vi "SaveParameters.vi"(9 "JSON_Text":string, 11 "ShiftConfigPath":path) -> ()   [LabVIEW 2017]
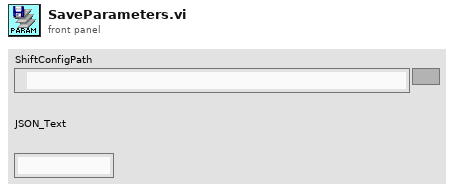
[diagram p1: front panel]
types:
  T1 = enum16{"open", "replace", "create", "open or create", "replace or create", "replace or create with confirmation"}
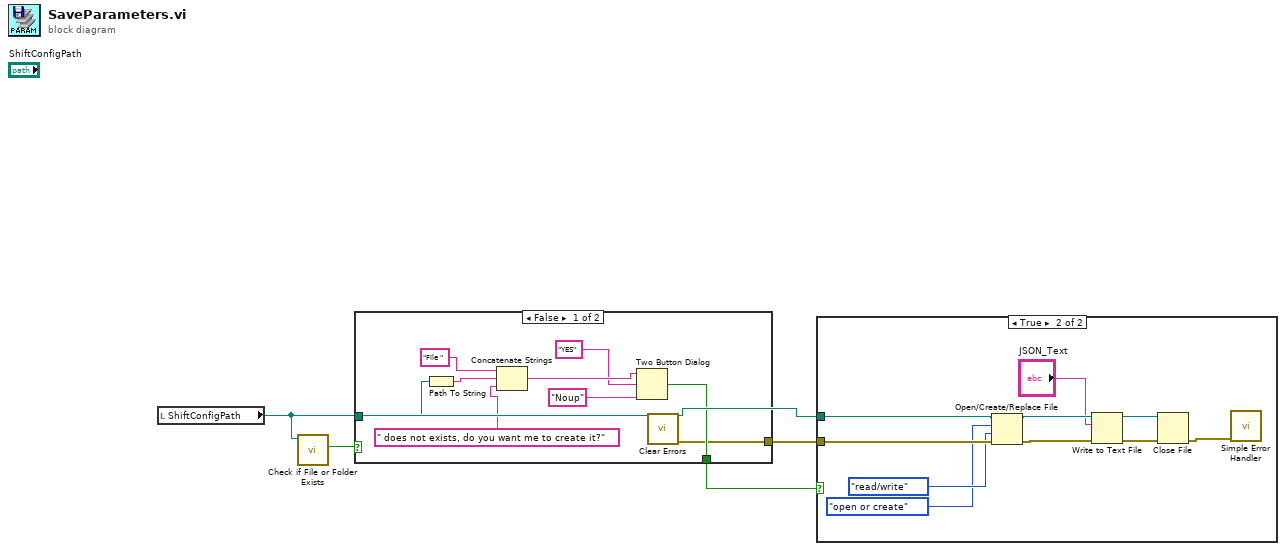
[diagram p0: block diagram]
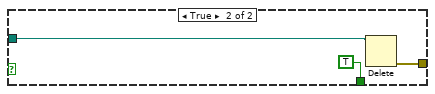
[diagram p3: hidden frame]
diagram:
  n1 = local read "ShiftConfigPath"() -> (w3:path)
  n2 = call <vilib>:"Check if File or Folder Exists.vi"("path"=w3) -> ("file or folder exists?"=w2:bool)  [unwired: 8 in, 2 out]
  n3 = case shown="False" w2 {
    tunnel: w3 -> [w13 w16]
    tunnel: [w5 w15] -> w4
    tunnel: [w6 TRUE] -> w1
    frame False {
      n4 = Path To String(path=w13) -> (string=w11:string)
      n5 = Concatenate Strings("File " ("message"), w11, " does not exists, do you want me to create it?" ("message")) -> (w9:string)
      n6 = Two Button Dialog(message=w9, 1:"Noup" ("T button name (\"OK\")"), 2:"YES" ("T button name (\"OK\")")) -> (T button?=w6:bool)
      n7 = call <vilib>:"Clear Errors.vi"() -> ("error out"=w5:errorcluster)  [unwired: 6 in, 1 out]
    }
    frame True {
      n8 = Delete(path (use dialog)=w16) -> (error out=w15:errorcluster)  [unwired: 4 in, 2 out]
    }
  }
  n9 = case shown="True" w1 {
    tunnel: w4 -> [_ w23]
    tunnel: w3 -> [_ w17]
    frame False {
    }
    frame True {
      n10 = Open/Create/Replace File(file path (use dialog)=w17, error in=w23, operation (0:open)=T1."open or create", access (0:read/write)=enum16{"read/write", "read-only", "write-only"}."read/write") -> (refnum out=w19:refnum<file>, error out=w20:errorcluster)  [unwired: 2 in, 1 out]
      n11 = Write to Text File(file (use dialog)=w19, text="JSON_Text", error in=w20) -> (refnum out=w25:refnum<file>, error out=w26:errorcluster)  [unwired: 1 in, 1 out]
      n12 = Close File(refnum=w25, error in=w26) -> (error out=w24:errorcluster)  [unwired: 1 out]
      n13 = call <vilib>:"Simple Error Handler.vi"("error in (no error)"=w24) -> ()  [unwired: 4 in, 5 out]
    }
  }
